vi "resultsColumnsTandP.vi"(10 "chValuesIn":string[](array[string]), 11 "chNamesIn":string[](array[string])) -> (2 "chValuesOut":string[](array[string]), 3 "chNamesOut":string[](array[string]))   [LabVIEW 2020]
uses:
  Globals/Meas_global.vi
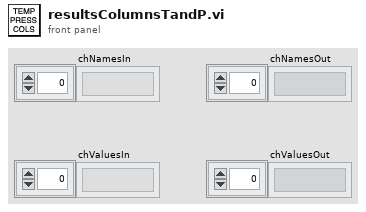
[diagram p1: front panel]
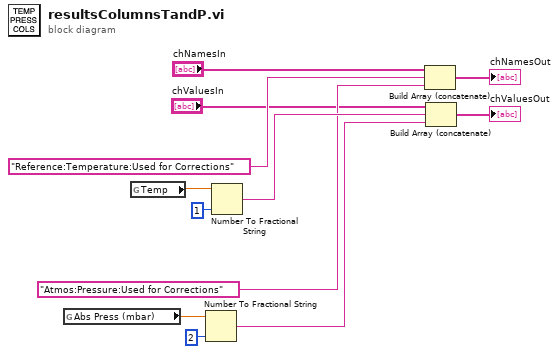
[diagram p0: block diagram]
diagram:
  n1 = global read "Meas_global.vi" "Abs Press (mbar)"() -> (w1:dbl)
  n2 = global read "Meas_global.vi" "Temp"() -> (w4:dbl)
  n3 = Number To Fractional String(number=w1, precision (6)=i16 2) -> (F-format string=w10:string)  [unwired: 2 out]
  n4 = Number To Fractional String(number=w4, precision (6)=i16 1) -> (F-format string=w9:string)  [unwired: 2 out]
  n5 = Build Array (concatenate)("chNamesIn", "Reference:Temperature:Used for Corrections", "Atmos:Pressure:Used for Corrections") -> (→"chNamesOut":string[])
  n6 = Build Array (concatenate)("chValuesIn", w9, w10) -> (→"chValuesOut":string[])
